vi "CVT to JSON Core.vi"(8 "error in (no error)":errorcluster, 10 "StrIn":string="{", 11 "variant":variant) -> (0 "error out":errorcluster, 2 "StrOut":string, 3 "Variant":variant)   [LabVIEW 2014]
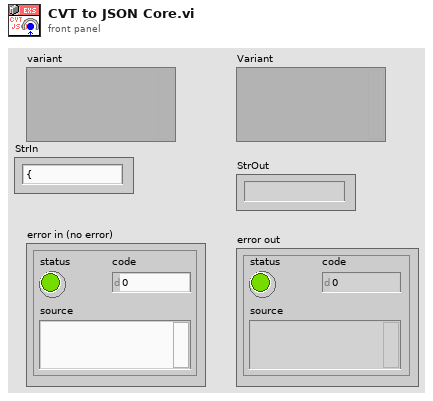
[diagram p1: front panel]
types:
  T1 = typedef "Type Descriptor Enumeration__ogtk.ctl" = enum8{"<Null>", "I8", "I16", "I32", "I64", "U8", "U16", "U32", "U64", "SGL", "DBL", "EXT", "CSG", "CDB", "CXT", "0x0F", "0x10", "0x11", "0x12", "0x13", "0x14", "Enum U8", "Enum U16", "Enum U32", "Enum U64", "SGL PQ", "DBL PQ", "EXT PQ", "CSG PQ", "CDB PQ", "CXT PQ", "0x1F", "0x20", "Boolean", "0x22", "0x23", "0x24", "0x25", "0x26", "0x27", "0x28", "0x29", "0x2A", "0x2B", "0x2C", "0x2D", "0x2E", "0x2F", "String", "0x31", "Path", "Pict", "0x34", "0x35", "0x36", "DAQ", "0x38", "0x39", "0x3A", "0x3B", "0x3C", "0x3D", "0x3E", "0x3F", "Array", "0x41", "0x42", "0x43", "0x44", "0x45", "0x46", "0x47", "0x48", "0x49", "0x4A", "0x4B", "0x4C", "0x4D", "0x4E", "0x4F", "Cluster", "0x51", "0x52", "Variant", "Waveform", "0x55", "0x56", "0x57", "0x58", "0x59", "0x5A", "0x5B", "0x5C", "0x5D", "0x5E", "0x5F", "0x60", "0x61", "0x62", "0x63", "0x64", "0x65", "0x66", "0x67", "0x68", "0x69", "0x6A", "0x6B", "0x6C", "0x6D", "0x6E", "0x6F", "Refnum"}
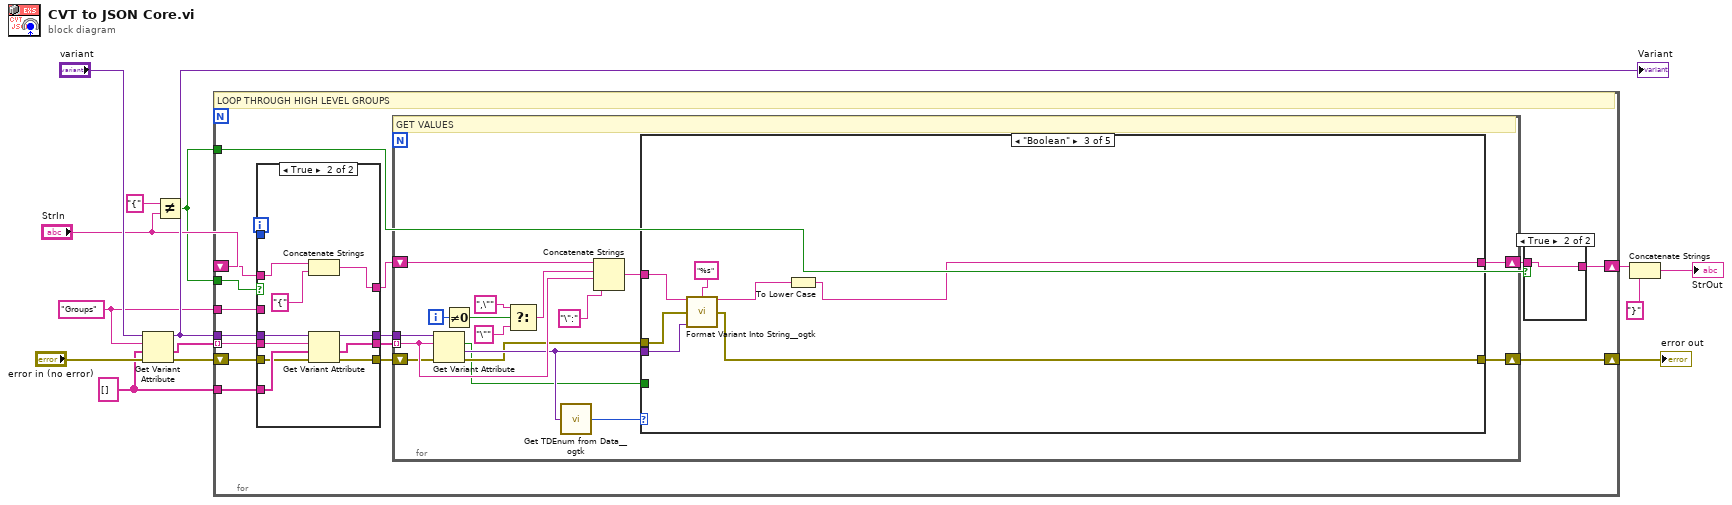
[diagram p0: block diagram]
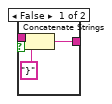
[diagram p2: hidden frame]
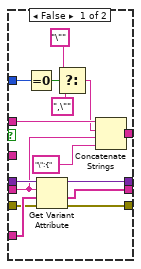
[diagram p3: hidden frame]
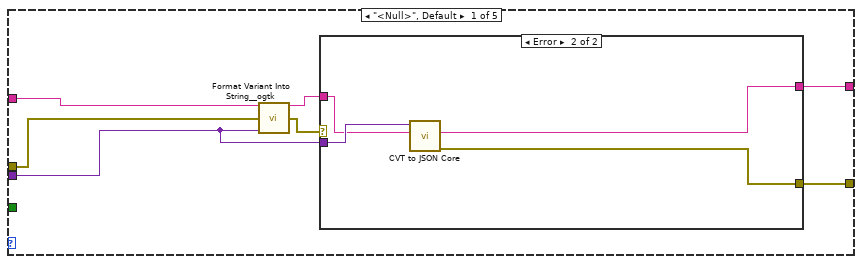
[diagram p4: hidden frame]
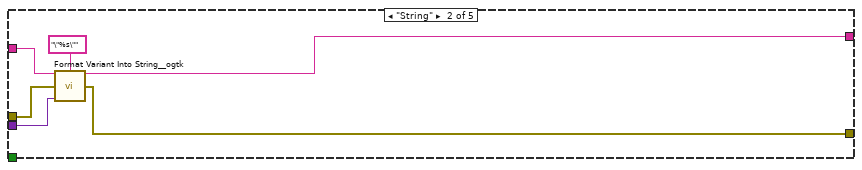
[diagram p6: hidden frame]
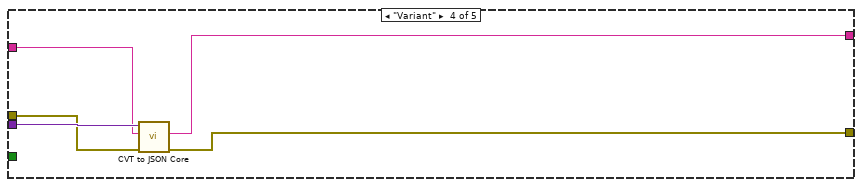
[diagram p7: hidden frame]
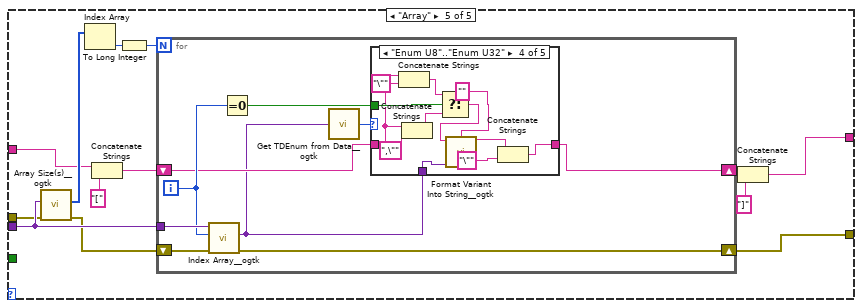
[diagram p8: hidden frame]
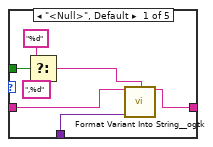
[diagram p9: hidden frame]
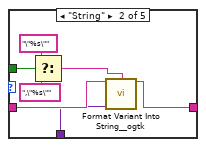
[diagram p10: hidden frame]
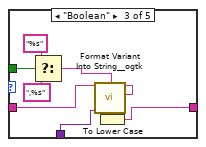
[diagram p11: hidden frame]
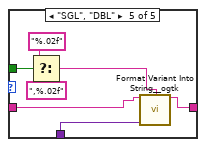
[diagram p12: hidden frame]
diagram:
  w7 = string[] []
  w2 = "Groups" ("name")
  n1 = Get Variant Attribute(Variant="variant", name=w2, default value (empty Variant)=w7, error in="error in (no error)") -> (duplicate Variant=w10:variant, value=w6:string[], error out=w13:errorcluster)  [unwired: 1 out]
  "Variant" <- w10
  n2 = Not Equal?(x="{", y="StrIn") -> (x != y?=w1:bool)
  n3 = for {
    tunnel: w10 -> [w30]
    tunnel: w6 -> [w25] mode=indexing
    tunnel: w7 -> [w29]
    shift-right: [w21] -> w8
    shift-left: "StrIn" -> [w26]
    shift-right: [w18] -> w14
    shift-left: w13 -> [w20]
    tunnel: w1 -> [w17]
    tunnel: w2 -> [w16]
    tunnel: w1 -> [w15]
    i -> [w23]
    # "LOOP THROUGH HIGH LEVEL GROUPS"
    n4 = case shown="True" w17 {
      tunnel: w30 -> [w49 w59]
      tunnel: w29 -> [w48 w57]
      tunnel: [w47 w54] -> w28
      tunnel: [w46 w58] -> w27
      tunnel: w26 -> [w45 w52]
      tunnel: w25 -> [w44 w53]
      tunnel: [w42 w50] -> w24
      tunnel: w23 -> [w41 _]
      tunnel: w20 -> [w36 w56]
      tunnel: [w35 w55] -> w19
      tunnel: w16 -> [_ _]
      frame False {
        n5 = Equal To 0?(x=w41) -> (x = 0?=w40:bool)
        n6 = Get Variant Attribute(Variant=w49, name=w44, default value (empty Variant)=w48, error in=w36) -> (duplicate Variant=w46:variant, value=w47:string[], error out=w35:errorcluster)  [unwired: 1 out]
        n7 = Select(t="\"" ("string"), s=w40, f=",\"" ("string")) -> (s? t:f=w37:string)
        n8 = Concatenate Strings(w45, w37, w44, "\":{" ("string")) -> (w42:string)
      }
      frame True {
        n9 = Concatenate Strings(w52, "{" ("x")) -> (w50:string)
        n10 = Get Variant Attribute(Variant=w59, name=w53, default value (empty Variant)=w57, error in=w56) -> (duplicate Variant=w58:variant, value=w54:string[], error out=w55:errorcluster)  [unwired: 1 out]
      }
    }
    n11 = for {
      tunnel: w28 -> [w75] mode=indexing
      tunnel: w27 -> [w76]
      shift-right: [w65] -> w22
      shift-left: w24 -> [w73]
      shift-right: [w61] -> w18
      shift-left: w19 -> [w63]
      i -> [w72]
      # "GET VALUES"
      n12 = Get Variant Attribute(Variant=w76, name=w75, error in=w63) -> (found=w60:bool, value=w66:variant, error out=w62:errorcluster)  [unwired: 1 in, 1 out]
      n13 = Not Equal To 0?(x=w72) -> (x != 0?=w71:bool)
      n14 = Select(t=",\"" ("string"), s=w71, f="\"" ("string")) -> (s? t:f=w68:string)
      n15 = call <userlib>:"Get TDEnum from Data__ogtk.vi"("Data"=w66) -> ("Type Descriptor Enumeration"=w67:T1)  [unwired: 4 in]
      n16 = Concatenate Strings(w73, w68, w75, "\":" ("string")) -> (w64:string)
      n17 = case shown="\"Boolean\"" w67 {
        tunnel: w66 -> [w79 w95 w102 w107 w113]
        tunnel: [w80 w92 w96 w105 w115] -> w65
        tunnel: w64 -> [w83 w93 w100 w103 w119]
        tunnel: w62 -> [w82 w90 w98 w106 w112]
        tunnel: [w77 w91 w99 w104 w110] -> w61
        tunnel: w60 -> [_ _ _ _ _]
        frame "<Null>", Default {
          n18 = call <userlib>:"Format Variant Into String__ogtk.vi"("Input String"=w83, "error in (no error)"=w82, "Variant"=w79) -> ("Output String"=w81:string, "error out"=w78:errorcluster)  [unwired: 11 in]
          n19 = case shown="Error" w78 {
            selector: w78 -> [w84 _]
            tunnel: w81 -> [w85 w87]
            tunnel: [w85 w86] -> w80
            tunnel: w79 -> [_ w89]
            tunnel: [w84 w88] -> w77
            frame No Error {
            }
            frame Error {
              n20 = call "CVT to JSON Core.vi"("StrIn"=w87, "variant"=w89) -> ("error out"=w88:errorcluster, "StrOut"=w86:string)  [unwired: 7 in, 1 out]
            }
          }
        }
        frame "String" {
          n21 = call <userlib>:"Format Variant Into String__ogtk.vi"("Input String"=w93, "Format String"="\"%s\"", "error in (no error)"=w90, "Variant"=w95) -> ("Output String"=w92:string, "error out"=w91:errorcluster)  [unwired: 10 in]
        }
        frame "Boolean" {
          n22 = call <userlib>:"Format Variant Into String__ogtk.vi"("Input String"=w100, "Format String"="%s", "error in (no error)"=w98, "Variant"=w102) -> ("Output String"=w97:string, "error out"=w99:errorcluster)  [unwired: 10 in]
          n23 = To Lower Case(string=w97) -> (all lower case string=w96:string)
        }
        frame "Variant" {
          n24 = call "CVT to JSON Core.vi"("error in (no error)"=w106, "StrIn"=w103, "variant"=w107) -> ("error out"=w104:errorcluster, "StrOut"=w105:string)  [unwired: 6 in, 1 out]
        }
        frame "Array" {
          n25 = call <userlib>:"Array Size(s)__ogtk.vi"("error in (no error)"=w112, "Array"=w113) -> ("error out"=w111:errorcluster, "Size(s)"=w120:u32[])  [unwired: 7 in, 1 out]
          n26 = Index Array(array=w120) -> (element=w109:u32)  [unwired: 1 in]
          n27 = Concatenate Strings(w119, "[" ("string")) -> (w117:string)
          n28 = To Long Integer(number=w109) -> (32bit integer=w108:i32)
          n29 = for {
            N: w108 -> [_]
            tunnel: w113 -> [w129]
            shift-right: [w122] -> w116
            shift-left: w117 -> [w123]
            shift-right: [w124] -> w110
            shift-left: w111 -> [w125]
            i -> [w128]
            n30 = call <userlib>:"Index Array__ogtk.vi"("error in (no error)"=w125, "Index (1D)"=w128, "MultiD Array"=w129) -> ("error out"=w124:errorcluster, "Array Element"=w121:variant)  [unwired: 7 in]
            n31 = Equal To 0?(x=w128) -> (x = 0?=w127:bool)
            n32 = call <userlib>:"Get TDEnum from Data__ogtk.vi"("Data"=w121) -> ("Type Descriptor Enumeration"=w126:T1)  [unwired: 4 in]
            n33 = case shown="\"Enum U8\"..\"Enum U32\"" w126 {
              tunnel: w127 -> [w134 w141 w149 w163 w170]
              tunnel: w123 -> [w132 w139 w147 w159 w166]
              tunnel: [w130 w137 w146 w153 w164] -> w122
              tunnel: w121 -> [w131 w138 w144 w152 w165]
              frame "<Null>", Default {
                n34 = Select(t="%d", s=w134, f=",%d") -> (s? t:f=w133:string)
                n35 = call <userlib>:"Format Variant Into String__ogtk.vi"("Input String"=w132, "Format String"=w133, "Variant"=w131) -> ("Output String"=w130:string)  [unwired: 11 in, 1 out]
              }
              frame "String" {
                n36 = Select(t="\"%s\"", s=w141, f=",\"%s\"") -> (s? t:f=w140:string)
                n37 = call <userlib>:"Format Variant Into String__ogtk.vi"("Input String"=w139, "Format String"=w140, "Variant"=w138) -> ("Output String"=w137:string)  [unwired: 11 in, 1 out]
              }
              frame "Boolean" {
                n38 = Select(t="%s", s=w149, f=",%s") -> (s? t:f=w148:string)
                n39 = call <userlib>:"Format Variant Into String__ogtk.vi"("Input String"=w147, "Format String"=w148, "Variant"=w144) -> ("Output String"=w145:string)  [unwired: 11 in, 1 out]
                n40 = To Lower Case(string=w145) -> (all lower case string=w146:string)
              }
              frame "Enum U8".."Enum U32" {
                n41 = Concatenate Strings(w159, "\"" ("string")) -> (w160:string)
                n42 = Concatenate Strings(w159, ",\"" ("string")) -> (w161:string)
                n43 = Select(t=w160, s=w163, f=w161) -> (s? t:f=w156:string)
                n44 = call <userlib>:"Format Variant Into String__ogtk.vi"("Input String"=w156, "Format String"="", "Variant"=w152) -> ("Output String"=w154:string)  [unwired: 11 in, 1 out]
                n45 = Concatenate Strings(w154, "\"" ("string")) -> (w153:string)
              }
              frame "SGL", "DBL" {
                n46 = Select(t="%.02f", s=w170, f=",%.02f") -> (s? t:f=w167:string)
                n47 = call <userlib>:"Format Variant Into String__ogtk.vi"("Input String"=w166, "Format String"=w167, "Variant"=w165) -> ("Output String"=w164:string)  [unwired: 11 in, 1 out]
              }
            }
          }
          n48 = Concatenate Strings(w116, "]" ("string")) -> (w115:string)
        }
      }
    }
    n49 = case shown="True" w15 {
      tunnel: w22 -> [w33 w34]
      tunnel: [w31 w34] -> w21
      frame False {
        n50 = Concatenate Strings(w33, "}" ("string")) -> (w31:string)
      }
      frame True {
      }
    }
  }
  "error out" <- w14
  n51 = Concatenate Strings(w8, "}" ("string")) -> (→"StrOut":string)
